vi "GenerateCode.vi"(1 "Terms":T1[](array[typedef]), 3 "Diagram":refnum<vi>, 5 "XRef":refnum<vi>, 6 "State In":T4={"Input Type"=variant(dbl 0.0), "Width"=0, "Typedef Name"="", "Value Type"=variant, "Selection"=0, "Options"=[], "Selections"=[], "Display Selections"=[], "Element Names"=[], "Typedef Name Width"=0, "Display Selection Width"=[], "Code Generated"=FALSE}) -> (0 "Generated Code?":bool, 2 "State Out":T4={"Input Type"=variant(dbl 0.0), "Width"=0, "Typedef Name"="", "Value Type"=variant, "Selection"=0, "Options"=[], "Selections"=[], "Display Selections"=[], "Element Names"=[], "Typedef Name Width"=0, "Display Selection Width"=[], "Code Generated"=FALSE}, 4 "Reply":string[](array[string]))   [LabVIEW 2015, in "Read-Write-Signals.xnode"]
doc: "This ability VI is called when it is time to define the execution behavior of your XNode via LabVIEW's scripting API. This VI is only called when you have previously informed LabVIEW that you need to script through a GenerateCode reply. Diagram is a reference to a diagram of a temporary VI. This diagram contains exactly one front panel terminal for each terminal of your XNode. Terms is an array of pairs of Term IDs and terminal references. LabVIEW will copy code scripted into this diagram into your XNode and connect everything to the correct terminals. The front panel terminals that are on this diagram are special in that they can only be on the top level diagram.\n \n Generate Code? is used to tell LabVIEW whether or not you want to copy the scripted diagram over. If there is an error and you wish not to commit the changes, then the old XNode behavior will be left unchanged. If you set Generate Code? to false, then this VI will be called again next time type propagation is run. Otherwise, it will not be called until you indicate that it should be through the reply on another ability VI.\n \n Because the diagram you are scripting into is separate from the VI containing the XNode instance, type propagation and the data manager will run on the temporary VI after each scripting call.\n \n You should not use the Copy scripting method to move code into the temporary VI. This will adversely affect the user's clipboard. You should use the Move scripting method instead.\n\nDefault behavior: None.\n\nThis ability does not provide UI and OS messages are not handled.\n\nSee also: ModifyCode"
uses:
  Read-Write-Signals.xnode
  State.ctl
  Read-Write-Signals Item.ctl
  Read-Write-Signals Sub Item.ctl
  Read-Write-Signals Sub Item Type.ctl
  Read-Write-Signals Selection.ctl
  Read-Write-Signals Display Selection.ctl
  <vilib>/XNodeSupport/XNodeTermIDPair.ctl
  <vilib>/XNodeSupport/XNodeTermRef.ctl
  <vilib>/XNodeSupport/XNodeString.ctl
  <vilib>/LV-Scripting/LV-Scripting.lvlib
  <vilib>/Utility/Data Type/NI_Data Type.lvlib
  <vilib>/XNodeSupport/NI_XNodeSupport.lvlib
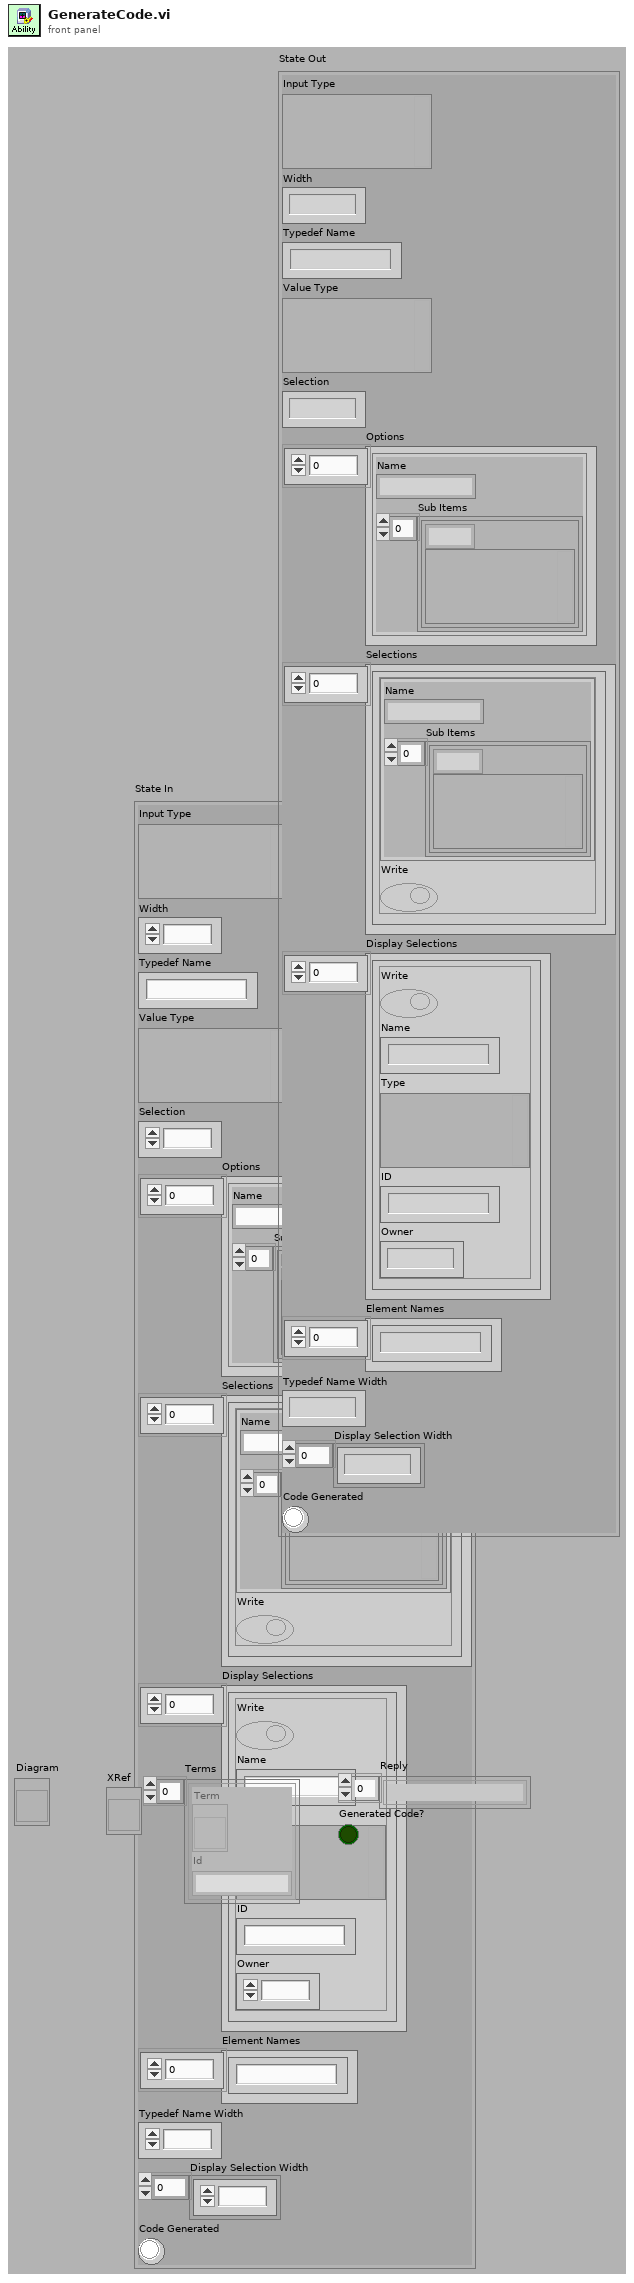
[diagram p1: front panel]
types:
  T1 = typedef "NI_XNodeSupport.lvlib/XNodeTermIDPair.ctl" = cluster{"Term":T2, "Id":T3}
  T2 = typedef "NI_XNodeSupport.lvlib/XNodeTermRef.ctl" = refnum<vi>
  T3 = typedef "NI_XNodeSupport.lvlib/XNodeString.ctl" = string
  T4 = typedef "Read-Write-Signals.xnode/State.ctl" = cluster{"Input Type":variant, "Width":i32, "Typedef Name":string, "Value Type":variant, "Selection":i32, "Options":T5[], "Selections":T8[], "Display Selections":T9[], "Element Names":string[], "Typedef Name Width":i32, "Display Selection Width":i32[], "Code Generated":bool}
  T5 = typedef "Read-Write-Signals Item.ctl" = cluster{"Name":string, "Sub Items":T6[]}
  T6 = typedef "Read-Write-Signals Sub Item.ctl" = cluster{"Type":T7, "Value":variant}
  T7 = typedef "Read-Write-Signals Sub Item Type.ctl" = enum8{"Cluster Element", "Array Element", "Subarray"}
  T8 = typedef "Read-Write-Signals Selection.ctl" = cluster{"Item":T5, "Write":bool}
  T9 = typedef "Read-Write-Signals Display Selection.ctl" = cluster{"Write":bool, "Name":string, "Type":variant, "ID":string, "Owner":i32}
  T10 = typedef "NI_Data Type.lvlib/Data Type.ctl" = enum8{"Invalid Type", "Void", "I8", "I16", "I32", "I64", "U8", "U16", "U32", "U64", "Single Float", "Double Float", "Extended Float", "Single Complex", "Double Complex", "Extended Complex", "Enum U8", "Enum U16", "Enum U32", "Enum U64", "Single Float With Unit", "Double Float With Unit", "Extended Float With Unit", "Single Complex with Unit", "Double Complex with Unit", "Extended Complex with Unit", "Boolean", "String", "Path", "Picture", "Tag", "Array", "Cluster", "Variant", "LV Variant", "Waveform", "Timestamp", "Digital Waveform", "Digital Data", "ExpressData", "Refnum", "External Data", "VI", "Poly VI", "LabVIEW Class Instance", "Fixed Point"}
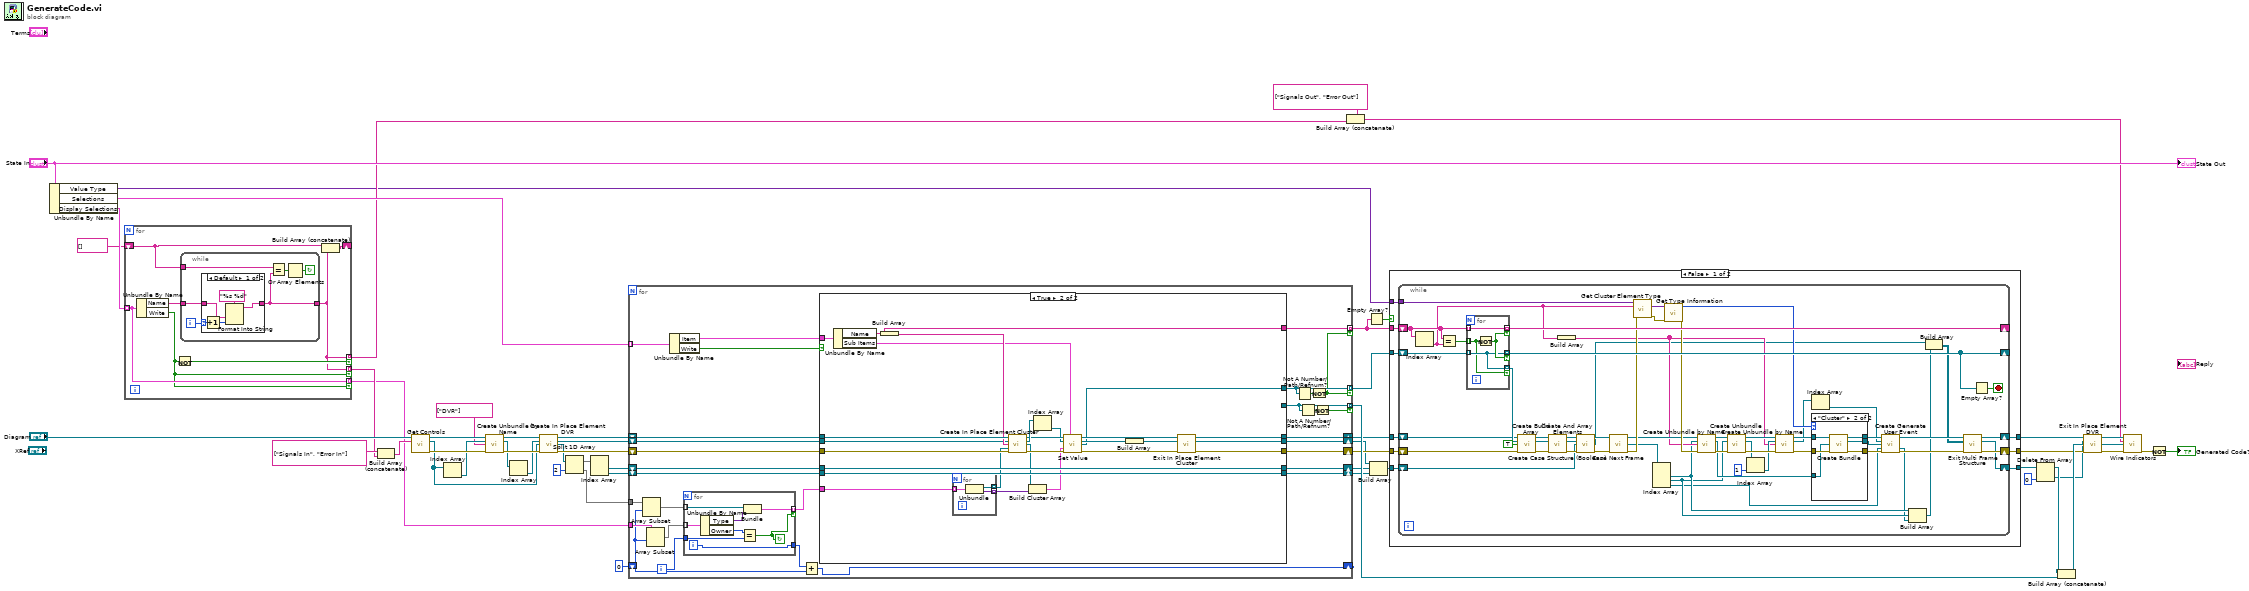
[diagram p0: block diagram]
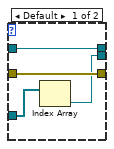
[diagram p2: hidden frame]
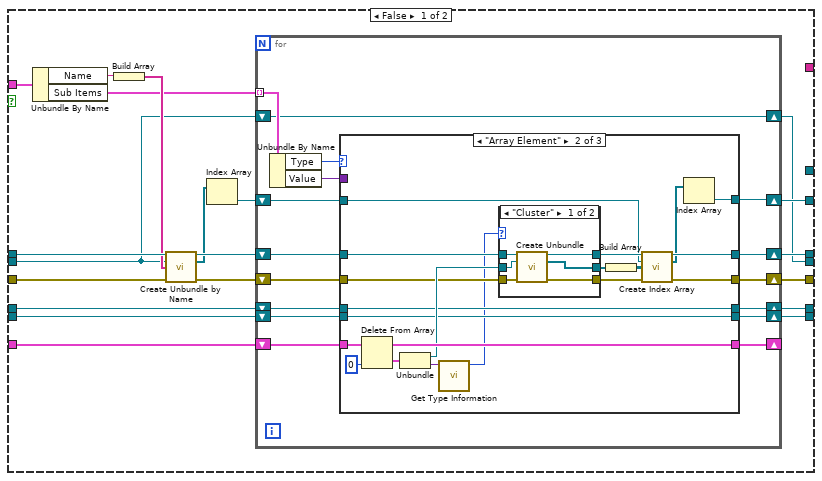
[diagram p4: hidden frame]
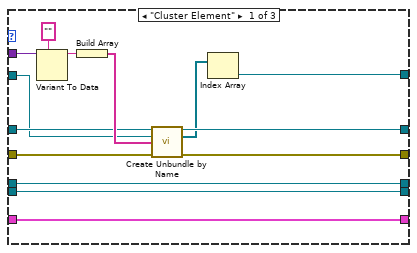
[diagram p5: hidden frame]
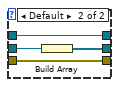
[diagram p6: hidden frame]
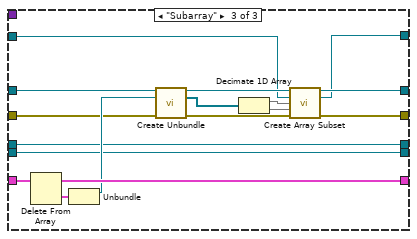
[diagram p7: hidden frame]
diagram:
  n1 = Unbundle By Name("State In") -> ("Value Type"=w16:variant, "Selections"=w41:T8[], "Display Selections"=w31:T9[])
  n2 = for {
    tunnel: w31 -> [w56] mode=indexing
    tunnel: [w57] -> w26 mode=indexing if=w61
    tunnel: [w57] -> w51 mode=indexing if=w55
    tunnel: [w56] -> w2 mode=indexing if=w55
    shift-right: [w60] -> _
    shift-left: string[] [] -> [w59]
    n3 = Unbundle By Name(w56) -> ("Name"=w58:string, "Write"=w55:bool)
    n4 = Not(x=w55) -> (.not. x?=w61:bool)
    n5 = while {
      tunnel: w58 -> [w65]
      tunnel: w59 -> [w67]
      tunnel: [w62] -> w57
      i -> [w66]
      stop <- w63 continue-if-true
      n6 = case shown="Default" w66 {
        selector: w66 -> [w71 _]
        tunnel: w65 -> [w70 w73]
        tunnel: [w69 w73] -> w62
        frame Default {
          n7 = Increment(x=w71) -> (x+1=w68:i32)
          n8 = Format Into String(format string="%s %d", w70, w68) -> (resulting string=w69:string)  [unwired: 2 in, 1 out]
        }
        frame 0 {
        }
      }
      n9 = Equal?(x=w67, y=w62) -> (x = y?=w64:bool[])
      n10 = Or Array Elements(Boolean array=w64) -> (logical OR=w63:bool)
    }
    n11 = Build Array (concatenate)(w59, w57) -> (w60:string[])
  }
  n12 = Build Array (concatenate)(string[] ["Signals In", "Error In"] ("Control Names"), w51) -> (w50:string[])
  n13 = call <vilib>:"Get Controls.vi"("Diagram in"="Diagram", "Control Names"=w50) -> ("Diagram out"=w49:refnum<vi>, "Control Terminals"=w35:refnum<vi>[], "error out"=w48:errorcluster)  [unwired: 11 in]
  n14 = Index Array(array=w35) -> (element=w47:refnum<vi>)  [unwired: 1 in]
  n15 = call <vilib>:"Create Unbundle by Name.vi"("Diagram in"=w49, "input cluster"=w47, "Element Names"=string[] ["DVR"], "error in (no error)"=w48) -> ("Diagram out"=w45:refnum<vi>, "Outputs"=w43:refnum<vi>[], "error out"=w44:errorcluster)  [unwired: 9 in]
  n16 = Index Array(array=w43) -> (element=w42:refnum<vi>)  [unwired: 1 in]
  n17 = call <vilib>:"Create In Place Element DVR.vi"("Diagram in"=w45, "DVR"=w42, "Inputs"=w35, "error in (no error)"=w44) -> ("Diagram out"=w40:refnum<vi>, "Data Value"=w38:refnum<vi>, "Inputs"=w33:refnum<vi>[], "error out"=w39:errorcluster)  [unwired: 7 in, 1 out]
  n18 = Split 1D Array(array=w33, index=2) -> (first subarray=w32:refnum<vi>[], second subarray=w3:refnum<vi>[])
  n19 = Index Array(array=w32) -> (element #1=w36:refnum<vi>, element #2=w37:refnum<vi>)  [unwired: 2 in]
  n20 = for {
    tunnel: w41 -> [w100] mode=indexing
    shift-right: [w94] -> w17
    shift-left: w40 -> [w99]
    shift-right: [w93] -> w18
    shift-left: w39 -> [w98]
    shift-right: [w91] -> w14
    shift-left: w37 -> [w95]
    shift-right: [w92] -> w15
    shift-left: w36 -> [w96]
    tunnel: [w88] -> w30 mode=indexing if=w89
    shift-right: [w87] -> w13
    shift-left: w38 -> [w97]
    tunnel: [w85] -> w19 mode=indexing if=w83
    tunnel: [w84] -> w21 mode=indexing if=w83
    tunnel: w3 -> [w78]
    tunnel: w2 -> [w80]
    shift-right: [w76] -> _
    shift-left: 0 -> [w74]
    i -> [w82]
    n21 = Array Subset(array=w78, index=w74) -> (w77:refnum<vi>[])  [unwired: 1 in]
    n22 = Array Subset(array=w80, index=w74) -> (w79:T9[])  [unwired: 1 in]
    n23 = Unbundle By Name(w100) -> ("Item"=w101:T5, "Write"=w102:bool)
    n24 = for {
      tunnel: w77 -> [w106] mode=indexing
      tunnel: w79 -> [w110] mode=indexing
      tunnel: w82 -> [w108]
      tunnel: [w105] -> w81 mode=indexing if=w104
      tunnel: [w103] -> w75
      i -> [w103]
      stop <- w104 continue-if-true
      n25 = Unbundle By Name(w110) -> ("Type"=w107:variant, "Owner"=w109:i32)
      n26 = Equal?(x=w109, y=w108) -> (x = y?=w104:bool)
      n27 = Bundle(w106, "Type"=w107) -> (w105:cluster{refnum<vi>, "Type":variant})  [unwired: 1 in]
    }
    n28 = Add(x=w75, y=w74) -> (x+y=w76:i32)
    n29 = case shown="True" w102 {
      tunnel: w101 -> [w130 w233]
      tunnel: w99 -> [w129 w231]
      tunnel: w98 -> [w126 w229]
      tunnel: w97 -> [w112 w226]
      tunnel: w81 -> [w120 w213]
      tunnel: w96 -> [w119 w215]
      tunnel: w95 -> [w118 w216]
      tunnel: [w117 w224] -> w94
      tunnel: [w116 w225] -> w93
      tunnel: [w115 w215] -> w92
      tunnel: [w114 w216] -> w91
      tunnel: [w113 _] -> w88
      tunnel: [w111 w223] -> w87
      tunnel: [_ w209] -> w85
      tunnel: [_ w208] -> w84
      frame False {
        n30 = Unbundle By Name(w130) -> ("Name"=w128:string, "Sub Items"=w125:T6[])
        n31 = Build Array(w128) -> (w127:string[])
        n32 = call <vilib>:"Create Unbundle by Name.vi"("Diagram in"=w129, "input cluster"=w112, "Element Names"=w127, "error in (no error)"=w126) -> ("Diagram out"=w124:refnum<vi>, "Outputs"=w122:refnum<vi>[], "error out"=w123:errorcluster)  [unwired: 9 in]
        n33 = Index Array(array=w122) -> (element=w121:refnum<vi>)  [unwired: 1 in]
        n34 = for {
          tunnel: w125 -> [w146] mode=indexing
          shift-right: [w136] -> _
          shift-left: w120 -> [w143]
          shift-right: [w135] -> w117
          shift-left: w124 -> [w142]
          shift-right: [w134] -> w116
          shift-left: w123 -> [w141]
          shift-right: [w138] -> w115
          shift-left: w119 -> [w139]
          shift-right: [w137] -> w114
          shift-left: w118 -> [w140]
          shift-right: [w132] -> w113
          shift-left: w121 -> [w133]
          shift-right: [w131] -> w111
          shift-left: w112 -> [w131]
          n35 = Unbundle By Name(w146) -> ("Type"=w145:T7, "Value"=w144:variant)
          n36 = case shown="\"Array Element\"" w145 {
            tunnel: w144 -> [w158 _ _]
            tunnel: w143 -> [w147 w180 w207]
            tunnel: w142 -> [w154 w176 w203]
            tunnel: w141 -> [w153 w175 w202]
            tunnel: w140 -> [w159 w165 w201]
            tunnel: w139 -> [w160 w164 w200]
            tunnel: [w160 w164 w200] -> w138
            tunnel: [w159 w165 w201] -> w137
            tunnel: [w147 w179 w206] -> w136
            tunnel: [w152 w173 w197] -> w135
            tunnel: [w151 w172 w198] -> w134
            tunnel: w133 -> [w150 w168 w194]
            tunnel: [w148 w166 w196] -> w132
            frame "Cluster Element" {
              n37 = Variant To Data(type="", Variant=w158) -> (data=w156:string)  [unwired: 1 in, 1 out]
              n38 = Build Array(w156) -> (w155:string[])
              n39 = call <vilib>:"Create Unbundle by Name.vi"("Diagram in"=w154, "input cluster"=w150, "Element Names"=w155, "error in (no error)"=w153) -> ("Diagram out"=w152:refnum<vi>, "Outputs"=w149:refnum<vi>[], "error out"=w151:errorcluster)  [unwired: 9 in]
              n40 = Index Array(array=w149) -> (element=w148:refnum<vi>)  [unwired: 1 in]
            }
            frame "Array Element" {
              n41 = Delete From Array(array=w180, index=0) -> (deleted portion=w178:cluster{refnum<vi>, "Type":variant}, array with subset deleted=w179:cluster{refnum<vi>, "Type":variant}[])  [unwired: 1 in]
              n42 = Unbundle(w178) -> (w177:refnum<vi>, "Type"=w163:variant)
              n43 = call <vilib>:"Get Type Information.vi"("Variant"=w163) -> ("Type"=w162:T10)  [unwired: 6 in, 4 out]
              n44 = case shown="\"Cluster\"" w162 {
                tunnel: w177 -> [w184 w190]
                tunnel: w176 -> [w186 w188]
                tunnel: w175 -> [w185 w189]
                tunnel: [w182 w189] -> w171
                tunnel: [w183 w188] -> w170
                tunnel: [w181 w187] -> w169
                frame "Cluster" {
                  n45 = call <vilib>:"Create Unbundle.vi"("Diagram in"=w186, "input cluster"=w184, "error in (no error)"=w185) -> ("Diagram out"=w183:refnum<vi>, "Outputs"=w181:refnum<vi>[], "error out"=w182:errorcluster)  [unwired: 10 in]
                }
                frame Default {
                  n46 = Build Array(w190) -> (w187:refnum<vi>[])
                }
              }
              n47 = Build Array(w169) -> (w174:refnum<vi>[][])
              n48 = call <vilib>:"Create Index Array.vi"("Diagram in"=w170, "array"=w168, "Indices"=w174, "error in (no error)"=w171) -> ("Diagram out"=w173:refnum<vi>, "Outputs"=w167:refnum<vi>[], "error out"=w172:errorcluster)  [unwired: 9 in]
              n49 = Index Array(array=w167) -> (element=w166:refnum<vi>)  [unwired: 1 in]
            }
            frame "Subarray" {
              n50 = Delete From Array(array=w207) -> (deleted portion=w205:cluster{refnum<vi>, "Type":variant}, array with subset deleted=w206:cluster{refnum<vi>, "Type":variant}[])  [unwired: 2 in]
              n51 = Unbundle(w205) -> (w204:refnum<vi>)  [unwired: 1 out]
              n52 = call <vilib>:"Create Unbundle.vi"("Diagram in"=w203, "input cluster"=w204, "error in (no error)"=w202) -> ("Diagram out"=w195:refnum<vi>, "Outputs"=w193:refnum<vi>[], "error out"=w199:errorcluster)  [unwired: 10 in]
              n53 = Decimate 1D Array(w193) -> (w192:refnum<vi>[], w191:refnum<vi>[])
              n54 = call <vilib>:"Create Array Subset.vi"("Diagram in"=w195, "array"=w194, "Indices"=w192, "Lengths"=w191, "error in (no error)"=w199) -> ("Diagram out"=w197:refnum<vi>, "subarray"=w196:refnum<vi>, "error out"=w198:errorcluster)  [unwired: 8 in]
            }
          }
        }
      }
      frame True {
        n55 = Unbundle By Name(w233) -> ("Name"=w208:string, "Sub Items"=w222:T6[])
        n56 = Build Array(w208) -> (w227:string[])
        n57 = for {
          tunnel: w213 -> [w236] mode=indexing
          tunnel: [w235] -> w212 mode=indexing
          tunnel: [w234] -> w214 mode=indexing
          n58 = Unbundle(w236) -> (w235:refnum<vi>, "Type"=w234:variant)
        }
        n59 = call <vilib>:"Create In Place Element Cluster.vi"("Diagram in"=w231, "Cluster"=w226, "Element Names"=w227, "Inputs"=w212, "error in (no error)"=w229) -> ("Diagram out"=w221:refnum<vi>, "Elements"=w228:refnum<vi>[], "Inputs"=w211:refnum<vi>[], "error out"=w230:errorcluster)  [unwired: 7 in]
        n60 = Build Cluster Array(w211, w214) -> (w210:cluster{refnum<vi>, "Type":variant}[])
        n61 = Index Array(array=w228) -> (element=w220:refnum<vi>)  [unwired: 1 in]
        n62 = call "Set Value.vi"("Diagram in"=w221, "Sub Items"=w222, "Value in"=w220, "Input Terms in"=w210, "error in (no error)"=w230) -> ("Diagram out"=w217:refnum<vi>, "Value out"=w219:refnum<vi>, "Equal"=w209:refnum<vi>, "error out"=w232:errorcluster)  [unwired: 6 in, 1 out]
        n63 = Build Array(w219) -> (w218:refnum<vi>[])
        n64 = call <vilib>:"Exit In Place Element Cluster.vi"("Diagram in"=w217, "Elements"=w218, "error in (no error)"=w232) -> ("Diagram out"=w224:refnum<vi>, "Cluster"=w223:refnum<vi>, "error out"=w225:errorcluster)  [unwired: 9 in, 1 out]
      }
    }
    n65 = Not A Number/Path/Refnum?(number/path/refnum=w85) -> (NaN/Path/Refnum?=w86:bool)
    n66 = Not A Number/Path/Refnum?(number/path/refnum=w88) -> (NaN/Path/Refnum?=w90:bool)
    n67 = Not(x=w86) -> (.not. x?=w83:bool)
    n68 = Not(x=w90) -> (.not. x?=w89:bool)
  }
  n69 = Build Array (concatenate)(string[] ["Signals Out", "Error Out"] ("Control Names"), w26) -> (w25:string[])
  n70 = Empty Array?(array=w21) -> (empty?=w20:bool)
  n71 = Build Array(w13, w15, w14) -> (w12:refnum<vi>[])
  n72 = case shown="False" w20 {
    tunnel: w21 -> [w245 _]
    tunnel: w19 -> [w244 _]
    tunnel: w18 -> [w243 w317]
    tunnel: w17 -> [w242 w316]
    tunnel: w12 -> [w241 w318]
    tunnel: w16 -> [w240 _]
    tunnel: [w239 w318] -> w9
    tunnel: [w238 w316] -> w11
    tunnel: [w237 w317] -> w10
    frame False {
      n73 = while {
        shift-right: [w299] -> _
        shift-left: w245 -> [w300]
        shift-right: [w296] -> _
        shift-left: w244 -> [w298]
        shift-right: [w257] -> w237
        shift-left: w243 -> [w293]
        shift-right: [w247] -> w238
        shift-left: w242 -> [w286]
        shift-right: [w248] -> w239
        shift-left: w241 -> [w249]
        tunnel: w240 -> [w285]
        stop <- w297 stop-if-true
        n74 = Index Array(array=w300) -> (element=w274:string)  [unwired: 1 in]
        n75 = Equal?(x=w300, y=w274) -> (x = y?=w301:bool[])
        n76 = for {
          tunnel: w301 -> [w312] mode=indexing
          tunnel: w300 -> [w315] mode=indexing
          tunnel: [w315] -> w299 mode=indexing if=w314
          tunnel: w298 -> [w313] mode=indexing
          tunnel: [w313] -> w296 mode=indexing if=w314
          tunnel: [w313] -> w295 mode=indexing if=w312
          n77 = Not(x=w312) -> (.not. x?=w314:bool)
        }
        n78 = call <vilib>:"Create Build Array.vi"("Diagram in"=w286, "Inputs"=w295, "Concatenate Inputs"=TRUE, "error in (no error)"=w293) -> ("Diagram out"=w290:refnum<vi>, "appended array"=w289:refnum<vi>, "error out"=w292:errorcluster)  [unwired: 9 in]
        n79 = call <vilib>:"Create And Array Elements.vi"("Diagram in"=w290, "Boolean array"=w289, "error in (no error)"=w292) -> ("Diagram out"=w288:refnum<vi>, "logical AND"=w287:refnum<vi>, "error out"=w291:errorcluster)  [unwired: 10 in]
        n80 = Build Array(w274) -> (w265:string[])
        n81 = call <vilib>:"Create Case Structure (Boolean).vi"("Diagram in"=w288, "Selector"=w287, "Inputs"=w249, "error in (no error)"=w291) -> ("Selected Diagram"=w277:refnum<vi>, "Inputs"=w252:refnum<vi>[], "error out"=w284:errorcluster)  [unwired: 8 in, 1 out]
        n82 = call <vilib>:"Case Next Frame.vi"("Diagram in"=w277, "error in (no error)"=w284) -> ("Selected Diagram"=w276:refnum<vi>, "Inputs"=w275:refnum<vi>[], "error out"=w278:errorcluster)  [unwired: 10 in, 1 out]
        n83 = call <vilib>:"Get Cluster Element Type.vi"("error in (no error)"=w278, "Element Name"=w274, "Cluster in"=w285) -> ("error out"=w282:errorcluster, "Type"=w283:variant)  [unwired: 6 in, 1 out]
        n84 = Index Array(array=w275) -> (element #1=w255:refnum<vi>, element #2=w254:refnum<vi>, element #3=w253:refnum<vi>)  [unwired: 3 in]
        n85 = call <vilib>:"Get Type Information.vi"("error in (no error)"=w282, "Variant"=w283) -> ("error out"=w280:errorcluster, "Type"=w281:T10)  [unwired: 5 in, 3 out]
        n86 = call <vilib>:"Create Unbundle by Name.vi"("Diagram in"=w276, "input cluster"=w255, "Element Names"=w265, "error in (no error)"=w280) -> ("Diagram out"=w272:refnum<vi>, "Outputs"=w260:refnum<vi>[], "error out"=w273:errorcluster)  [unwired: 9 in]
        n87 = call <vilib>:"Create Unbundle.vi"("Diagram in"=w272, "input cluster"=w254, "error in (no error)"=w273) -> ("Diagram out"=w269:refnum<vi>, "Outputs"=w268:refnum<vi>[], "error out"=w271:errorcluster)  [unwired: 10 in]
        n88 = Index Array(array=w268, index=1) -> (element=w266:refnum<vi>)
        n89 = call <vilib>:"Create Unbundle by Name.vi"("Diagram in"=w269, "input cluster"=w266, "Element Names"=w265, "error in (no error)"=w271) -> ("Diagram out"=w264:refnum<vi>, "Outputs"=w259:refnum<vi>[], "error out"=w270:errorcluster)  [unwired: 9 in]
        n90 = case shown="\"Cluster\"" w281 {
          tunnel: w270 -> [w305 w311]
          tunnel: [w305 w310] -> w279
          tunnel: w264 -> [w304 w309]
          tunnel: [w304 w308] -> w262
          tunnel: [w303 w307] -> w261
          tunnel: w260 -> [w302 w306]
          frame Default {
            n91 = Index Array(array=w302) -> (element=w303:refnum<vi>)  [unwired: 1 in]
          }
          frame "Cluster" {
            n92 = call <vilib>:"Create Bundle.vi"("Diagram in"=w309, "Inputs"=w306, "error in (no error)"=w311) -> ("Diagram out"=w308:refnum<vi>, "output cluster"=w307:refnum<vi>, "error out"=w310:errorcluster)  [unwired: 10 in]
          }
        }
        n93 = Index Array(array=w259) -> (element=w258:refnum<vi>)  [unwired: 1 in]
        n94 = call <vilib>:"Create Generate User Event.vi"("Diagram in"=w262, "user event"=w258, "event data cluster"=w261, "error in"=w253, "error in (no error)"=w279) -> ("Diagram out"=w256:refnum<vi>, 10:"error out"=w246:refnum<vi>, 15:"error out"=w263:errorcluster)  [unwired: 7 in, 1 out]
        n95 = Build Array(w255, w254, w246) -> (w251:refnum<vi>[])
        n96 = Build Array(w252, w251) -> (w250:refnum<vi>[][])
        n97 = call <vilib>:"Exit Multi Frame Structure.vi"("Diagram in"=w256, "Outputs"=w250, "error in (no error)"=w263) -> ("Diagram out"=w247:refnum<vi>, "Outputs"=w248:refnum<vi>[], "error out"=w257:errorcluster)  [unwired: 10 in]
        n98 = Empty Array?(array=w296) -> (empty?=w297:bool)
      }
    }
    frame True {
    }
  }
  n99 = Delete From Array(array=w9, index=0) -> (deleted portion=w6:refnum<vi>, array with subset deleted=w8:refnum<vi>[])  [unwired: 1 in]
  n100 = Build Array (concatenate)(w8, w30) -> (w29:refnum<vi>[])
  n101 = call <vilib>:"Exit In Place Element DVR.vi"("Diagram in"=w11, "Data Value"=w6, "Outputs"=w29, "error in (no error)"=w10) -> ("Diagram out"=w28:refnum<vi>, "Outputs"=w24:refnum<vi>[], "error out"=w23:errorcluster)  [unwired: 7 in, 2 out]
  n102 = call <vilib>:"Wire Indicators.vi"("Diagram in"=w28, "Indicator Names"=w25, "Outputs"=w24, "error in (no error)"=w23) -> ("error out"=w4:errorcluster)  [unwired: 10 in, 1 out]
  n103 = Not(x=w4) -> (.not. x?=→"Generated Code?":bool)
  "State Out" <- "State In"
